vi "MecaDrivePoseEst_ResetPosition.vi"(9 "Gyro":T1={"VALUE"=0.0, "COS"=1.0, "SIN"=0.0} {"SIN" format="%13.4f"; "COS" format="%13.4f"; "VALUE" format="%13.4f"}, 10 "Pose":T10={"TRANSLATION"={"X"=0.0, "Y"=0.0}, "ROTATION"={"VALUE"=0.0, "COS"=1.0, "SIN"=0.0}} {"ROTATION"."SIN" format="%13.4f"; "ROTATION"."COS" format="%13.4f"; "ROTATION"."VALUE" format="%13.4f"; "TRANSLATION"."Y" format="%14.3f"; "TRANSLATION"."X" format="%14.3f"}, 11 "in MecaDrivePoseEstimate":T2={"M_VisionContR"=[], "m_nominal_dT"=0.0, "m_PrevTime_Sec"=0.0, "m_GyroOffset"={"VALUE"=0.0, "COS"=1.0, "SIN"=0.0}, "m_PrevAngle"={"VALUE"=0.0, "COS"=1.0, "SIN"=0.0}, "m_Observer"={"m_P"=[], "m_xHat"=[], "States"=0, "Outputs"=0, "m_ContR"=[], "m_ContQ"=[], "m_SigmasF"=[], "m_dT_Sec"=0.0, "MERWE_SCALED_SIGMA_PTS"={"m_Wm"=[], "States"=0, "Alpha"=0.0, "m_Wc"=[], "Kappa"=0}, "meanFuncX"=refnum, "meanFuncY"=refnum, "residualFuncX"=refnum, "residualFuncY"=refnum, "addFuncX"=refnum, "addFuncXExtra"=variant, "residualFuncYExtra"=variant, "residualFuncXExtra"=variant, "MeanFuncYExtra"=variant, "MeanFuncXExtra"=variant, "Inputs"=0}, "m_kinematics"={"FrontLeft"={"X"=0.0, "Y"=0.0}, "FrontRight"={"X"=0.0, "Y"=0.0}, "RearLeft"={"X"=0.0, "Y"=0.0}, "RearRight"={"X"=0.0, "Y"=0.0}, "InverseKinematics"=[[0.0, 1.0, -1.0, 0.0], [0.0, 1.0, 1.0, 0.0], [0.0, 1.0, 1.0, 0.0], [0.0, 1.0, -1.0, 0.0]], "ForwardKinematics"=[[0.0, 1.0, -1.0, 0.0], [0.0, 1.0, 1.0, 0.0], [0.0, 1.0, 1.0, 0.0], [0.0, 1.0, -1.0, 0.0]], "PrevCoR"={"X"=0.0, "Y"=0.0}}, "Pose_Buffer"={"TimeStamps"=[], "Pose"=[], "Min_TimeStamp"=0.0, "Max_TimeStamp"=0.0, "ItemCount"=0, "MaxBufferTime"=0.0}} {"Pose_Buffer"."Pose"."ROTATION"."SIN" format="%13.4f"; "Pose_Buffer"."Pose"."ROTATION"."COS" format="%13.4f"; "Pose_Buffer"."Pose"."ROTATION"."VALUE" format="%13.4f"; "Pose_Buffer"."Pose"."TRANSLATION"."Y" format="%14.3f"; "Pose_Buffer"."Pose"."TRANSLATION"."X" format="%14.3f"; "m_kinematics"."PrevCoR"."Y" format="%14.3f"; "m_kinematics"."PrevCoR"."X" format="%14.3f"; "m_kinematics"."RearRight"."Y" format="%14.3f"; "m_kinematics"."RearRight"."X" format="%14.3f"; "m_kinematics"."RearLeft"."Y" format="%14.3f"; "m_kinematics"."RearLeft"."X" format="%14.3f"; "m_kinematics"."FrontRight"."Y" format="%14.3f"; "m_kinematics"."FrontRight"."X" format="%14.3f"; "m_kinematics"."FrontLeft"."Y" format="%14.3f"; "m_kinematics"."FrontLeft"."X" format="%14.3f"; "m_PrevAngle"."SIN" format="%13.4f"; "m_PrevAngle"."COS" format="%13.4f"; "m_PrevAngle"."VALUE" format="%13.4f"; "m_GyroOffset"."SIN" format="%13.4f"; "m_GyroOffset"."COS" format="%13.4f"; "m_GyroOffset"."VALUE" format="%13.4f"}) -> (3 "Out PoseDrivePoseEstimate":T2={"M_VisionContR"=[], "m_nominal_dT"=0.0, "m_PrevTime_Sec"=0.0, "m_GyroOffset"={"VALUE"=0.0, "COS"=1.0, "SIN"=0.0}, "m_PrevAngle"={"VALUE"=0.0, "COS"=1.0, "SIN"=0.0}, "m_Observer"={"m_P"=[], "m_xHat"=[], "States"=0, "Outputs"=0, "m_ContR"=[], "m_ContQ"=[], "m_SigmasF"=[], "m_dT_Sec"=0.0, "MERWE_SCALED_SIGMA_PTS"={"m_Wm"=[], "States"=0, "Alpha"=0.0, "m_Wc"=[], "Kappa"=0}, "meanFuncX"=refnum, "meanFuncY"=refnum, "residualFuncX"=refnum, "residualFuncY"=refnum, "addFuncX"=refnum, "addFuncXExtra"=variant, "residualFuncYExtra"=variant, "residualFuncXExtra"=variant, "MeanFuncYExtra"=variant, "MeanFuncXExtra"=variant, "Inputs"=0}, "m_kinematics"={"FrontLeft"={"X"=0.0, "Y"=0.0}, "FrontRight"={"X"=0.0, "Y"=0.0}, "RearLeft"={"X"=0.0, "Y"=0.0}, "RearRight"={"X"=0.0, "Y"=0.0}, "InverseKinematics"=[[0.0, 1.0, -1.0, 0.0], [0.0, 1.0, 1.0, 0.0], [0.0, 1.0, 1.0, 0.0], [0.0, 1.0, -1.0, 0.0]], "ForwardKinematics"=[[0.0, 1.0, -1.0, 0.0], [0.0, 1.0, 1.0, 0.0], [0.0, 1.0, 1.0, 0.0], [0.0, 1.0, -1.0, 0.0]], "PrevCoR"={"X"=0.0, "Y"=0.0}}, "Pose_Buffer"={"TimeStamps"=[], "Pose"=[], "Min_TimeStamp"=0.0, "Max_TimeStamp"=0.0, "ItemCount"=0, "MaxBufferTime"=0.0}} {"Pose_Buffer"."Pose"."ROTATION"."SIN" format="%13.4f"; "Pose_Buffer"."Pose"."ROTATION"."COS" format="%13.4f"; "Pose_Buffer"."Pose"."ROTATION"."VALUE" format="%13.4f"; "Pose_Buffer"."Pose"."TRANSLATION"."Y" format="%14.3f"; "Pose_Buffer"."Pose"."TRANSLATION"."X" format="%14.3f"; "m_kinematics"."PrevCoR"."Y" format="%14.3f"; "m_kinematics"."PrevCoR"."X" format="%14.3f"; "m_kinematics"."RearRight"."Y" format="%14.3f"; "m_kinematics"."RearRight"."X" format="%14.3f"; "m_kinematics"."RearLeft"."Y" format="%14.3f"; "m_kinematics"."RearLeft"."X" format="%14.3f"; "m_kinematics"."FrontRight"."Y" format="%14.3f"; "m_kinematics"."FrontRight"."X" format="%14.3f"; "m_kinematics"."FrontLeft"."Y" format="%14.3f"; "m_kinematics"."FrontLeft"."X" format="%14.3f"; "m_PrevAngle"."SIN" format="%13.4f"; "m_PrevAngle"."COS" format="%13.4f"; "m_PrevAngle"."VALUE" format="%13.4f"; "m_GyroOffset"."SIN" format="%13.4f"; "m_GyroOffset"."COS" format="%13.4f"; "m_GyroOffset"."VALUE" format="%13.4f"})   [LabVIEW 2019, in "Trajectory_Library.lvlib"]
doc: "Resets the robot's position on the field.\n \n(NOTE -- For LabVIEW version, this may not be needed.) You NEED to reset your encoders (to zero) when calling this method.\n \nThe gyroscope angle does not need to be reset in the user's robot code. The library automatically takes care of offsetting the gyro angle.\n \nInputs:\n - SwervePoseEst -- Data cluster containing SwervePoseEst data\n - poseMeters -- The position on the field that your robot is at.\n - gyroAngle -- The angle reported by the gyroscope.\n\nOutputs:\n - outSwevePoseEst -- Updated data cluster"
uses:
  Trajectory_Library.lvlib
  MECA_DRIVE_POSE_EST.ctl
  <vilib>/Analysis/Matrix/Datatypes/RealMatrix.ctl
  ROTATION2D.ctl
  UNSCENTED_KALMAN_FILTER.ctl
  MERWE_SCALED_SIGMA_PTS.ctl
  CALLBACK_FUNC_TYPE.ctl
  MECA_DRIVE_KINEMATICS.ctl
  TRANSLATION2D.ctl
  TIME_INTERPOLATABLE_POSE2D.ctl
  POSE2D.ctl
  VecBuilder_3x1Fill.vi
  Pose2d_getXYAngle.vi
  Rotation2d_UnaryMinus.vi
  Rotation2d_RotateBy.vi
  MatBuilder_Create.vi
  Rotation2d_CreateAngle.vi
  Rotation2d_CreateXY.vi
  Util_CalcDist.vi
  <vilib>/Analysis/Matrix/NI_Matrix.lvlib
panel:
  # "<3, 3>"
  # "State Estimate <Statess,1>"
  # "<States, States>"
  # "<States, ?>"
  # "<Statess,  States>"
  # "<Outputs, Outputs>"
  # "<?, 1>"
  # "<?, 1>"
  # "<3, 3>"
  # "State Estimate <Statess,1>"
  # "<States, States>"
  # "<States, ?>"
  # "<Statess,  States>"
  # "<Outputs, Outputs>"
  # "<?, 1>"
  # "<?, 1>"
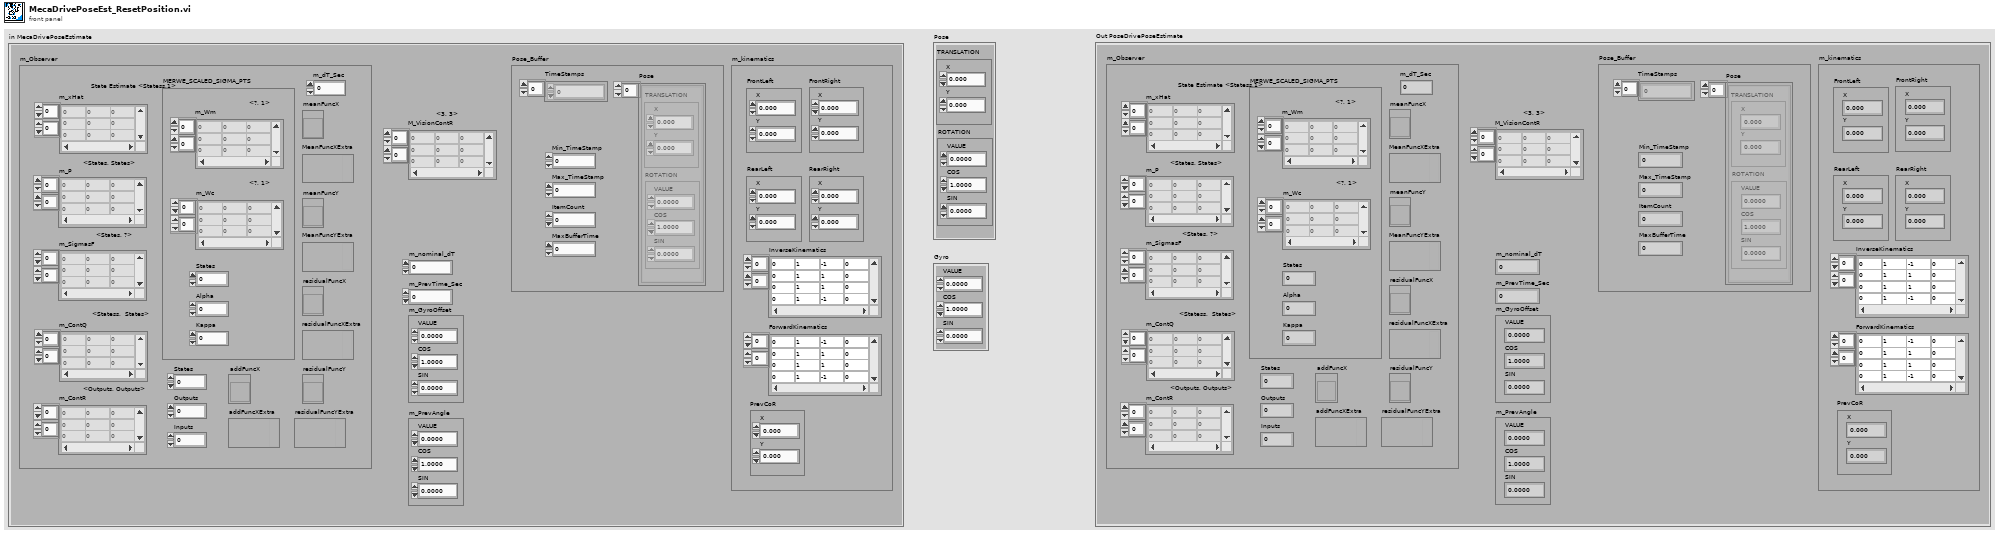
[diagram p1: front panel]
types:
  T1 = typedef "Trajectory_Library.lvlib/ROTATION2D.ctl" = cluster{"VALUE":dbl, "COS":dbl, "SIN":dbl}
  T2 = typedef "Trajectory_Library.lvlib/MECA_DRIVE_POSE_EST.ctl" = cluster{"M_VisionContR":T3, "m_nominal_dT":dbl, "m_PrevTime_Sec":dbl, "m_GyroOffset":T1, "m_PrevAngle":T1, "m_Observer":T4, "m_kinematics":T7, "Pose_Buffer":T9}
  T3 = typedef "NI_Matrix.lvlib/RealMatrix.ctl" = dbl[][]
  T4 = typedef "Trajectory_Library.lvlib/UNSCENTED_KALMAN_FILTER.ctl" = cluster{"m_P":T3, "m_xHat":T3, "States":i32, "Outputs":i32, "m_ContR":T3, "m_ContQ":T3, "m_SigmasF":T3, "m_dT_Sec":dbl, "MERWE_SCALED_SIGMA_PTS":T5, "meanFuncX":T6, "meanFuncY":T6, "residualFuncX":T6, "residualFuncY":T6, "addFuncX":T6, "addFuncXExtra":variant, "residualFuncYExtra":variant, "residualFuncXExtra":variant, "MeanFuncYExtra":variant, "MeanFuncXExtra":variant, "Inputs":i32}
  T5 = typedef "Trajectory_Library.lvlib/MERWE_SCALED_SIGMA_PTS.ctl" = cluster{"m_Wm":T3, "States":i32, "Alpha":dbl, "m_Wc":T3, "Kappa":i32}
  T6 = typedef "Trajectory_Library.lvlib/CALLBACK_FUNC_TYPE.ctl" = refnum<vi>
  T7 = typedef "Trajectory_Library.lvlib/MECA_DRIVE_KINEMATICS.ctl" = cluster{"FrontLeft":T8, "FrontRight":T8, "RearLeft":T8, "RearRight":T8, "InverseKinematics":T3, "ForwardKinematics":T3, "PrevCoR":T8}
  T8 = typedef "Trajectory_Library.lvlib/TRANSLATION2D.ctl" = cluster{"X":dbl, "Y":dbl}
  T9 = typedef "Trajectory_Library.lvlib/TIME_INTERPOLATABLE_POSE2D.ctl" = cluster{"TimeStamps":dbl[], "Pose":T10[], "Min_TimeStamp":dbl, "Max_TimeStamp":dbl, "ItemCount":i32, "MaxBufferTime":dbl}
  T10 = typedef "Trajectory_Library.lvlib/POSE2D.ctl" = cluster{"TRANSLATION":T8, "ROTATION":T1}
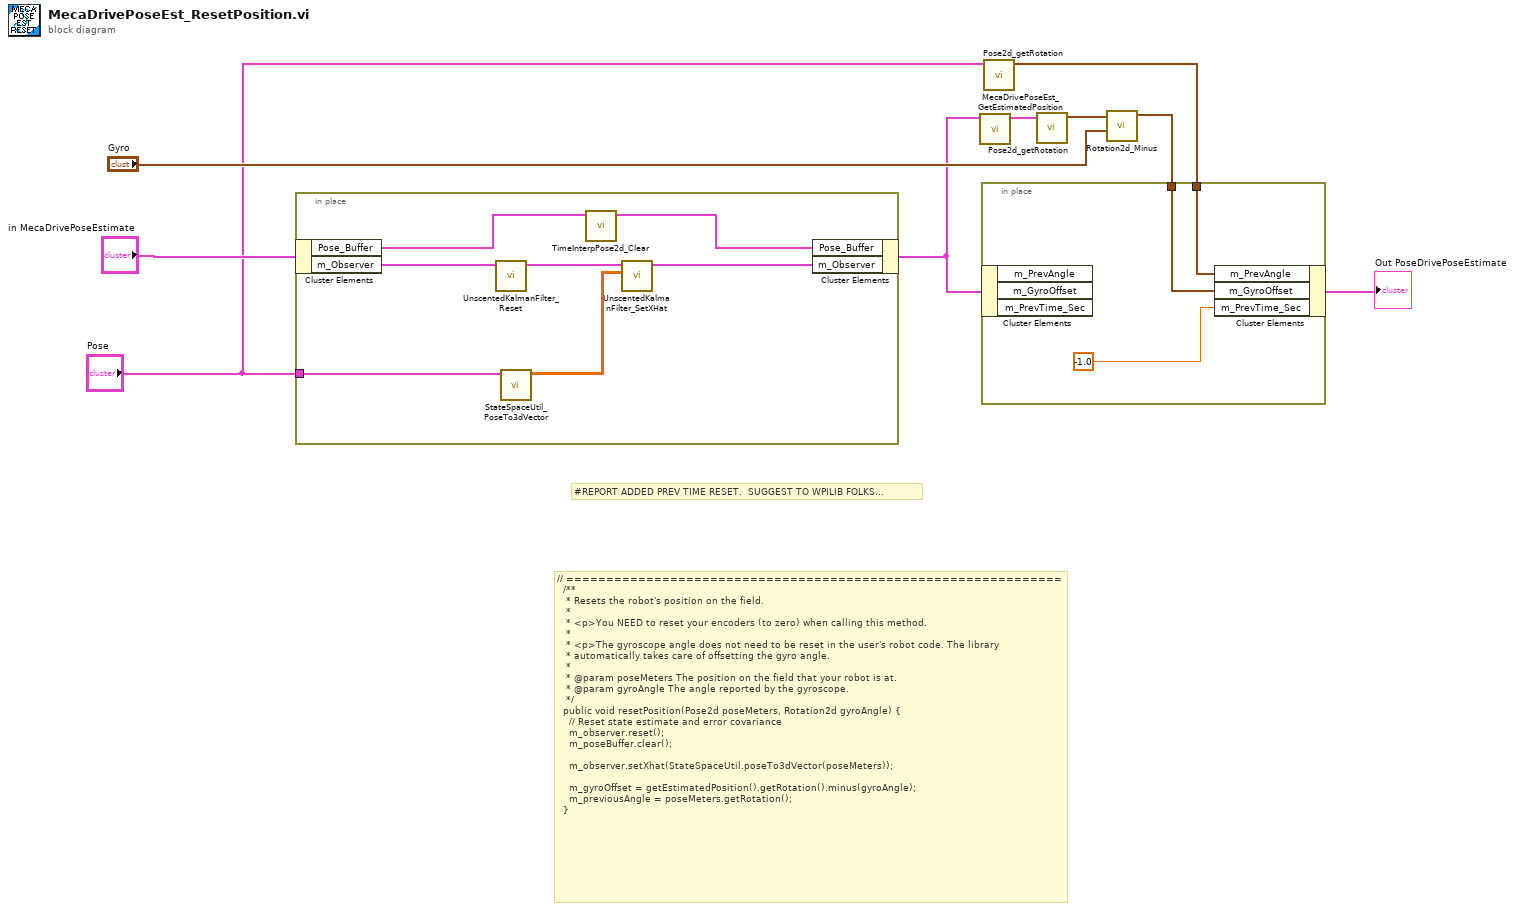
[diagram p0: block diagram]
diagram:
  # "// ==============================================================\n  /**\n   * Resets the robot's position on the field.\n   *\n   * <p>You NEED to reset your encoders (to zero) when calling this method.\n   *\n   * <p>The gyroscope angle does not need to be reset in the user's robot code. The library\n   * automatically takes care of offsetting the gyro angle.\n   *\n   * @param poseMeters The position on the field that your robot is at.\n   * @param gyroAngle The angle reported by the gyroscope.\n   */\n  public void resetPosition(Pose2d poseMeters, Rotation2d gyroAngle) {\n    // Reset state estimate and error covariance\n    m_observer.reset();\n    m_poseBuffer.clear();\n\n    m_observer.setXhat(StateSpaceUtil.poseTo3dVector(poseMeters));\n\n    m_gyroOffset = getEstimatedPosition().getRotation().minus(gyroAngle);\n    m_previousAngle = poseMeters.getRotation();\n  }"
  # "#REPORT ADDED PREV TIME RESET.  SUGGEST TO WPILIB FOLKS..."
  n1 = in-place {
    in-place-border: "Pose" -> [w13]
    n2 = in-place-cluster #1("in MecaDrivePoseEstimate") -> ("Pose_Buffer"=w11:T9, "m_Observer"=w15:T4)
    n3 = call "UnscentedKalmanFilter_Reset.vi"("in UnscentedKalmanFiilter"=w15) -> ("out UnscentedKalmanFiilter"=w16:T4)  [unwired: 10 in]
    n4 = call "StateSpaceUtil_PoseTo3dVector.vi"("Pose"=w13) -> ("Pose Vector"=w12:T3)  [unwired: 10 in]
    n5 = call "TimeInterpPose2d_Clear.vi"("in TimeInterpPose"=w11) -> ("out TimeInterpPose"=w10:T9)  [unwired: 10 in]
    n6 = call "UnscentedKalmanFilter_SetXHat.vi"("xHat"=w12, "in UnscentedKalmanFiilter"=w16) -> ("out UnscentedKalmanFiilter"=w14:T4)  [unwired: 8 in, 1 out]
    n7 = in-place-cluster #1("Pose_Buffer"=w10, "m_Observer"=w14) -> (w5:T2)
  }
  n8 = call "MecaDrivePoseEst_GetEstimatedPosition.vi"("in PoseDrivePoseEstimate"=w5) -> ("Estimated Pose"=w9:T10)  [unwired: 10 in]
  n9 = call "Pose2d_getRotation.vi"("in POSE"="Pose") -> ("out ROTATION"=w2:T1)  [unwired: 10 in]
  n10 = call "Pose2d_getRotation.vi"("in POSE"=w9) -> ("out ROTATION"=w7:T1)  [unwired: 10 in]
  n11 = call "Rotation2d_Minus.vi"("other ROTATION"="Gyro", "in ROTATION"=w7) -> ("out ROTATION"=w4:T1)  [unwired: 9 in]
  n12 = in-place {
    in-place-border: w4 -> [w18]
    in-place-border: w2 -> [w17]
    n13 = in-place-cluster #2(w5) -> ()  [unwired: 3 out]
    n14 = in-place-cluster #2("m_PrevAngle"=w17, "m_GyroOffset"=w18, "m_PrevTime_Sec"=-1.0) -> (→"Out PoseDrivePoseEstimate":T2)
  }
